vi "Set Hardware Settings.vi"(10 "Hardware Settings":T1, 11 "Model in":refnum<class "Model.lvclass">) -> (3 "Model out":refnum<class "Model.lvclass">)   [LabVIEW 2015, in "Model.lvclass"]
uses:
  Model.lvclass
  Typedefs/Hardware Settings.ctl
  Typedefs/Actuator Types.ctl
  Typedefs/Cylinder Types.ctl
  Model.lvclass/Model.ctl
  Typedefs/FAMT Typedefs.lvlib
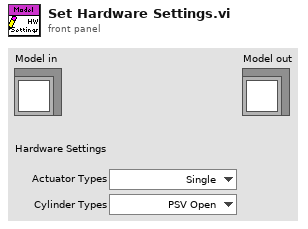
[diagram p1: front panel]
types:
  T1 = typedef "FAMT Typedefs.lvlib/Hardware Settings.ctl" = cluster{"Actuator Types":T2, "Cylinder Types":T3}
  T2 = typedef "FAMT Typedefs.lvlib/Actuator Types.ctl" = enum16{"Single", "Dual"}
  T3 = typedef "FAMT Typedefs.lvlib/Cylinder Types.ctl" = enum16{"PSV Open", "PSV Closed", "TV Open", "TV Closed", "Closed"}
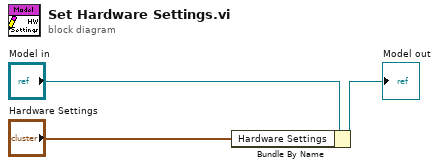
[diagram p0: block diagram]
diagram:
  n1 = Bundle By Name(cluster="Model in", "Hardware Settings"="Hardware Settings") -> (→"Model out":refnum<class "Model.lvclass">)
